vi "Drive Get Queue.vi"(8 "error in (no error)":errorcluster) -> (0 "error out":errorcluster, 3 "queue out":refnum<queue>)   [LabVIEW 2014]
uses:
  Action/Action.ctl
  Action/Action Priority.ctl
  Action/Action Name.ctl
  Action/Drive Action.ctl
  Action/Drive Action Name.ctl
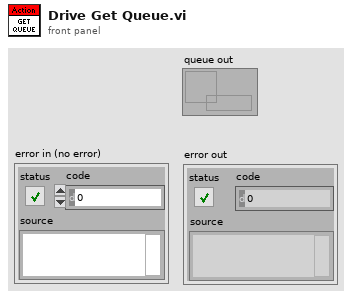
[diagram p1: front panel]
types:
  T1 = typedef "Drive Action.ctl" = cluster{"Priority":T2, "Name":T3, "Data":variant}
  T2 = typedef "Action Priority.ctl" = enum16{"Normal", "High", "Interrupt"}
  T3 = typedef "Drive Action Name.ctl" = enum16{"Left Drive", "Right Drive", "Half Drive", "Straight Drive"}
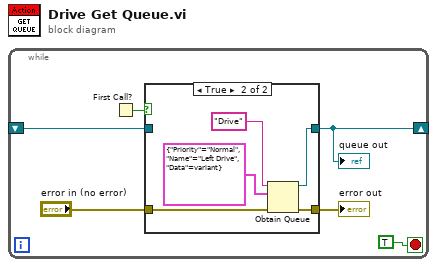
[diagram p0: block diagram]
diagram:
  n1 = while {
    shift-right: [w2] -> _
    shift-left: _ -> [w1]
    stop <- TRUE stop-if-true
    n2 = First Call?() -> (First Call?: T/F=w6:bool)
    n3 = case shown="True" w6 {
      tunnel: [w8 w11] -> w5
      tunnel: "error in (no error)" -> [w8 w10]
      tunnel: [w7 w9] -> w2
      tunnel: w1 -> [w7 _]
      frame False {
      }
      frame True {
        n4 = Obtain Queue(name (unnamed)="Drive", element data type=T1 {"Priority"=enum."Normal", "Name"=enum."Left Drive", "Data"=variant} ("Action"), error in (no error)=w10) -> (queue out=w9:refnum<queue>, error out=w11:errorcluster)  [unwired: 2 in, 1 out]
      }
    }
    "error out" <- w5
    "queue out" <- w2
  }
